vi "Global Settings.vi"() -> ()   [LabVIEW 2013, in "libssh2.lvlib"]
uses:
  libssh2.lvlib
panel:
  in  "Path":path
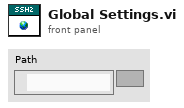
[diagram p1: front panel]
diagram:
